vi "Recordlog.vi"() -> ()   [LabVIEW 2020]
uses:
  <vilib>/Utility/file.llb/Write Delimited Spreadsheet (DBL).vi
  <vilib>/Utility/file.llb/Read Delimited Spreadsheet (string).vi
panel:
  in  "请输入账号":string caption="Please enter your account:"
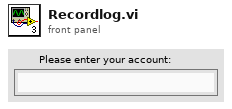
[diagram p1: front panel]
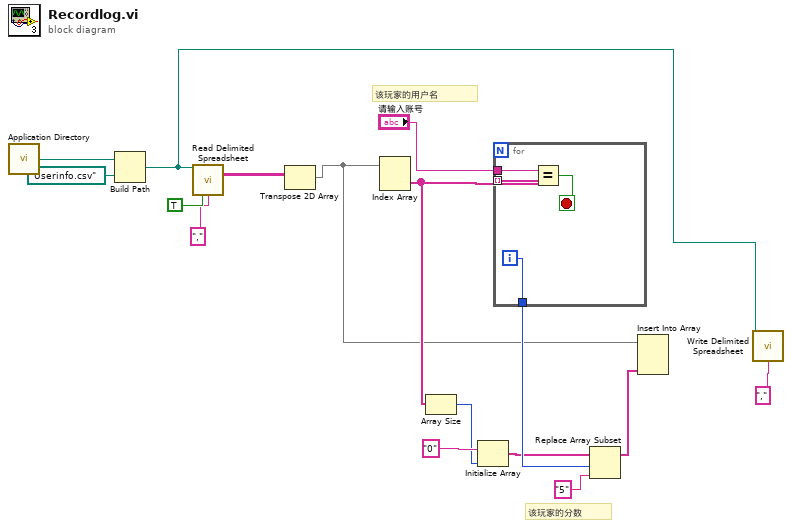
[diagram p0: block diagram]
diagram:
  # "该玩家的用户名"
  # "该玩家的分数"
  n1 = call <vilib>:"Application Directory.vi"() -> ("Application Directory"=w13:path)
  n2 = Build Path(base path=w13, name or relative path=path "Userinfo.csv") -> (appended path=w3:path)
  n3 = call-poly <vilib>:"Read Delimited Spreadsheet.vi"("file path (dialog if empty)"=w3, "transpose? (F)"=TRUE, "delimiter (\\t)"="," ("delimiter (\\t)")) -> ("all rows"=w12:string[][])  [unwired: 7 in, 5 out]
  n4 = Transpose 2D Array(2D array=w12) -> (transposed array=w1:string[][])
  n5 = Index Array(array=w1) -> (element=w8:string[])  [unwired: 2 in]
  n6 = Array Size(array=w8) -> (size(s)=w6:i32)
  n7 = Initialize Array("0", w6) -> (w5:string[])
  n8 = for {
    tunnel: "请输入账号" -> [w20]
    tunnel: w8 -> [w19] mode=indexing
    tunnel: [w17] -> w10
    i -> [w17]
    stop <- w18 stop-if-true
    n9 = Equal?(x=w20, y=w19) -> (x = y?=w18:bool)
  }
  n10 = Replace Array Subset(array=w5, new element="5", index=w10) -> (w2:string[])
  n11 = Insert Into Array(array=w1, new element=w2) -> ()  [unwired: 2 in, 1 out]
  n12 = call-poly <vilib>:"Write Delimited Spreadsheet.vi"("file path (dialog if empty)"=w3, "delimiter (\\t)"="," ("delimiter (\\t)")) -> ()  [unwired: 12 in, 2 out]
